vi "CRYUpdate CDD.vi"(9 "Document Data In":string, 10 "Flatten Data In":string, 11 "Signal":T1(ring)) -> (2 "Document Data Out":string, 3 "Flatten Data Out":string)   [LabVIEW 2013]
uses:
  CRYProject Editor Global.vi
  CRYSystem/Misc/SubVI/CRYMisc vis settings global.vi
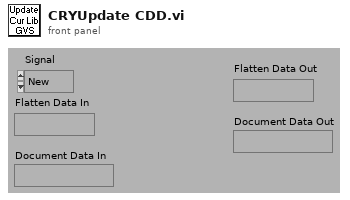
[diagram p1: front panel]
types:
  T1 = enum16{"New", "Open", "Close", "Close Data View Window Only", "Change", "Save", "Save for close"}
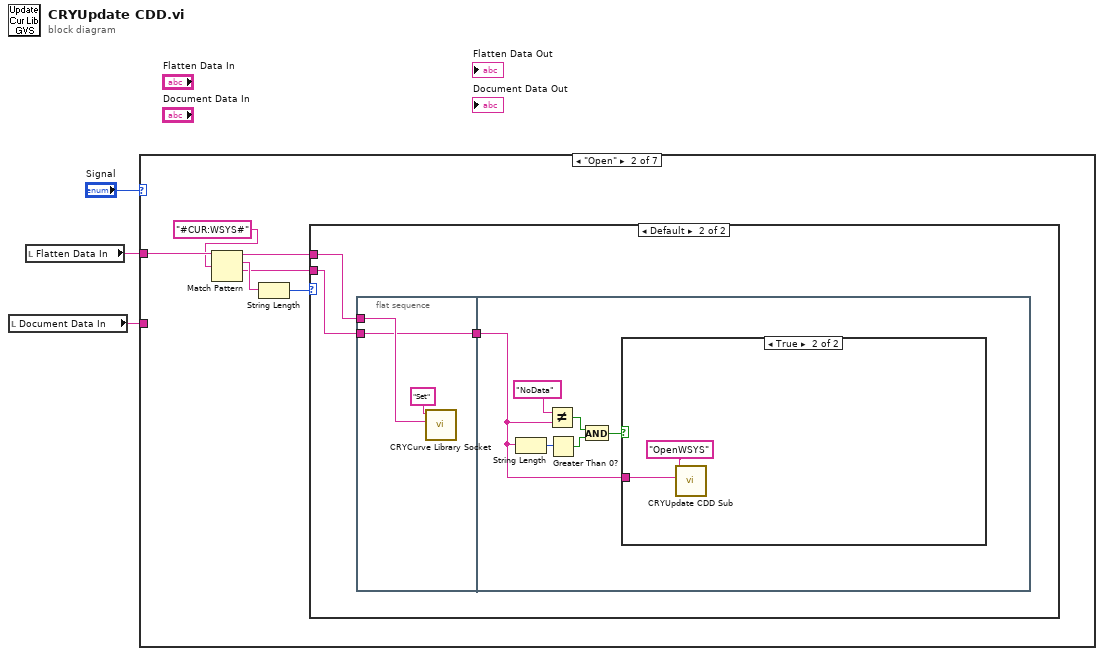
[diagram p0: block diagram]
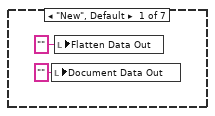
[diagram p2: hidden frame]
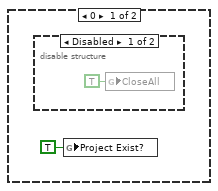
[diagram p3: hidden frame]
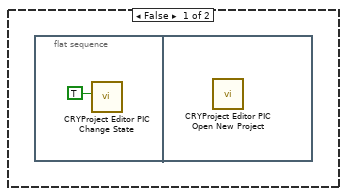
[diagram p5: hidden frame]
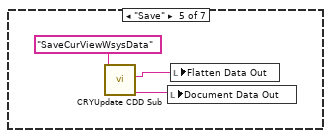
[diagram p8: hidden frame]
diagram:
  n1 = local read "Document Data In"() -> (w2:string)
  n2 = local read "Flatten Data In"() -> (w1:string)
  n3 = case shown="\"Open\"" "Signal" {
    tunnel: w1 -> [_ w11 _ _ _ _ _]
    tunnel: w2 -> [_ _ _ _ _ _ _]
    frame "New", Default {
      n4 = local write "Document Data Out"("" ("Document Data Out")) -> ()
      n5 = local write "Flatten Data Out"("" ("Flatten Data Out")) -> ()
    }
    frame "Open" {
      n6 = Match Pattern(string=w11, regular expression="#CUR:WSYS#") -> (before substring=w7:string, match substring=w9:string, after substring=w6:string)  [unwired: 1 in, 1 out]
      n7 = String Length(string=w9) -> (length=w8:i32)
      n8 = case shown="Default" w8 {
        tunnel: w7 -> [_ w16]
        tunnel: w6 -> [_ w15]
        frame 0 {
          n9 = disable-structure shown="Disabled" {
            frame Disabled {
              n10 = global write "CRYMisc vis settings global.vi" "CloseAll"(TRUE ("CloseAll")) -> ()
            }
            frame Enabled {
            }
          }
          n11 = global write "CRYProject Editor Global.vi" "Project Exist?"(TRUE ("Project Exist?")) -> ()
        }
        frame Default {
          n12 = flat-sequence {
            tunnel: w16 -> [w18]
            tunnel: w15 -> [w17]
            tunnel: [w17] -> w14
            tunnel: w14 -> [w20]
            frame #0 {
              n13 = call "CRYCurve Library Socket.vi"("sDataIn"=w18, "sAction"="Set") -> ()  [unwired: 9 in, 1 out]
            }
            frame #1 {
              n14 = String Length(string=w20) -> (length=w21:i32)
              n15 = Not Equal?(x="NoData", y=w20) -> (x != y?=w23:bool)
              n16 = Greater Than 0?(x=w21) -> (x > 0?=w24:bool)
              n17 = And(x=w23, y=w24) -> (x .and. y?=w25:bool)
              n18 = case shown="True" w25 {
                tunnel: w20 -> [_ w27]
                frame False {
                  n19 = flat-sequence {
                    frame #0 {
                      n20 = call "CRYProject Editor PIC Change State.vi"("bChangeState"=TRUE) -> ()  [unwired: 11 in]
                    }
                    frame #1 {
                      n21 = call "CRYProject Editor PIC Open New Project.vi"() -> ()  [unwired: 12 in]
                    }
                  }
                }
                frame True {
                  n22 = call "CRYUpdate CDD Sub.vi"("sData"=w27, "sAction"="OpenWSYS") -> ()  [unwired: 8 in, 2 out]
                }
              }
            }
          }
        }
      }
    }
    frame "Close Data View Window Only" {
    }
    frame "Change" {
    }
    frame "Save" {
      n23 = call "CRYUpdate CDD Sub.vi"("sAction"="SaveCurViewWsysData") -> ("Document Data Out"=w29:string, "Flatten Data Out"=w30:string)  [unwired: 9 in]
      n24 = local write "Document Data Out"(w29) -> ()
      n25 = local write "Flatten Data Out"(w30) -> ()
    }
    frame "Close" {
    }
    frame "Save for close" {
    }
  }
